vi "Database-CheckExist.vi"(8 "error in":errorcluster, 9 "Serial":string, 10 "Ref":string, 11 "System":string) -> (0 "error out":errorcluster, 1 "Repetitions":u8, 2 "Status":i8)   [LabVIEW 2016]
doc: "Go to DB->WriteStationValues action\nReturn boolean flag to show if data was saved to DB successfully\n\nWabco 2017 All right reserved\nAuthor: maciej.szupienko@wabco-auto.com"
uses:
  Database.Main.Action.ctl
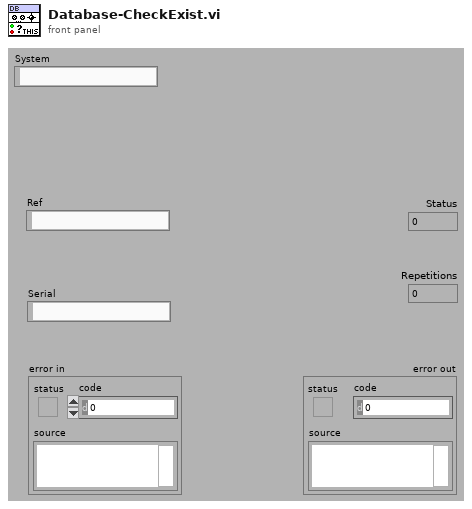
[diagram p1: front panel]
types:
  T1 = typedef "Database.Main.Action.ctl" = enum32{"idle", "constructor", "destructor", "--- DB ---", "Init", "Setup", "Select.Variant", "File.Export", "UpdateVariantFiles", "CheckStatus"}
  T2 = cluster{"System":string, "Ref":string, "Serial":string}
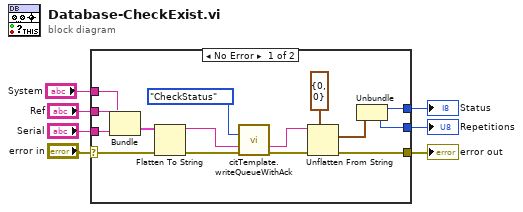
[diagram p0: block diagram]
diagram:
  n1 = case shown="No Error" "error in" {
    selector: "error in" -> [w21 w23]
    tunnel: [w19 w23] -> w6
    tunnel: [w11 _] -> w5
    tunnel: "Serial" -> [w16 _]
    tunnel: "Ref" -> [w15 _]
    tunnel: [w10 _] -> w2
    tunnel: "System" -> [w8 _]
    frame No Error {
      n2 = Bundle("System"=w8, "Ref"=w15, "Serial"=w16) -> (w17:T2)  [unwired: 1 in]
      n3 = Flatten To String(anything=w17, error in (no error)=w21) -> (data string=w14:string, error out=w20:errorcluster)  [unwired: 2 in, 1 out]
      n4 = call "citTemplate.writeQueueWithAck.vi"("event in"=Database.Main.Action."CheckStatus" ("Action"), "(flatten) data in"=w14, "error in (no error)"=w20) -> ("notification data"=w18:string, "error out"=w22:errorcluster)  [unwired: 10 in, 1 out]
      n5 = Unflatten From String(type=cluster{i8, u8} {0, 0}, binary string=w18, error in (no error)=w22) -> (value=w12:cluster{i8, u8}, error out=w19:errorcluster)  [unwired: 2 in, 1 out]
      n6 = Unbundle(w12) -> (w11:i8, w10:u8)
    }
    frame Error {
    }
  }
  "error out" <- w6
  "Status" <- w5
  "Repetitions" <- w2
